vi "Reset Timer.vi"(0 "reference in":refnum<class "Timer.lvclass">, 5 "error in (no error)":errorcluster) -> (14 "reference out":refnum<class "Timer.lvclass">, 19 "error out":errorcluster)   [LabVIEW 2017, in "Timer.lvclass"]
uses:
  Timer.lvclass
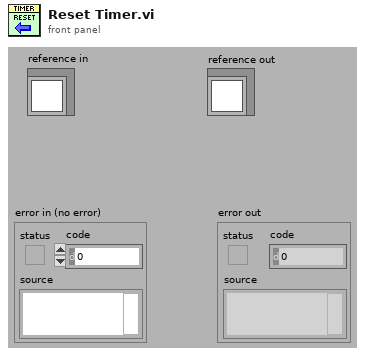
[diagram p1: front panel]
types:
  T1 = typedef "Timer.lvclass/ObjectAttributes.ctl" = cluster{"Timer is Timing":bool, "Timer Time (ms)":u32, "Timer VI Reference":refnum<vi>}
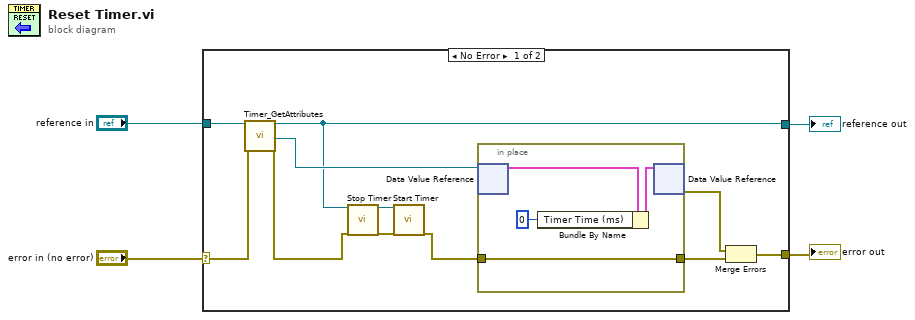
[diagram p0: block diagram]
diagram:
  n1 = case shown="No Error" "error in (no error)" {
    selector: "error in (no error)" -> [w14 w21]
    tunnel: [w12 w21] -> w3
    tunnel: [w6 w20] -> w1
    tunnel: "reference in" -> [w15 w20]
    frame No Error {
      n2 = call "Timer_GetAttributes.vi"("reference in"=w15, "error in (no error)"=w14) -> ("reference out"=w6:refnum<class "Timer.lvclass">, "DataRef"=w11:refnum<data-value>, "error out"=w9:errorcluster)  [unwired: 14 in, 1 out]
      n3 = call-dynamic "Stop Timer.vi"("reference in"=w6, "error in (no error)"=w9) -> ("reference out"=w5:refnum<class "Timer.lvclass">, "error out"=w8:errorcluster)  [unwired: 13 in, 3 out]
      n4 = call-dynamic "Start Timer.vi"("reference in"=w5, "error in (no error)"=w8) -> ("error out"=w7:errorcluster)  [unwired: 16 in, 1 out]
      n5 = in-place {
        in-place-border: w7 -> [w17]
        in-place-border: [w17] -> w10
        n6 = in-place-dvr #1(w11) -> (w18:T1)  [unwired: 1 out]
        n7 = Bundle By Name(cluster=w18, "Timer Time (ms)"=u32 0) -> (w19:T1)
        n8 = in-place-dvr #1(w19) -> (w13:errorcluster)  [unwired: 1 out]
      }
      n9 = Merge Errors(w13, w10) -> (w12:errorcluster)
    }
    frame Error {
    }
  }
  "error out" <- w3
  "reference out" <- w1
